vi "refnums.vi"() -> ()   [LabVIEW 2018]
panel:
  out "Wheel_1_Pot":string
  out "Wheel_4_Azimuth":string
  out "Wheel_3_Azimuth":string
  out "IMU_0":string
  out "Joystick_Driver":string
  out "Shifters":string
  out "Butterfly":string
  out "Compressor":string
  out "Wheel_2_Azimuth":string
  out "Wheel_1_Azimuth":string
  out "Wheel_4_Speed":string
  out "Wheel_3_Speed":string
  out "Wheel_2_Speed":string
  out "Wheel_1_Speed":string
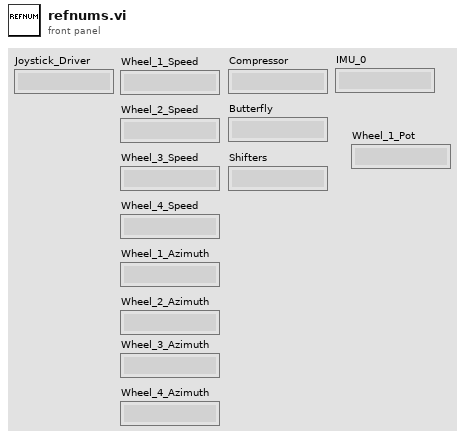
[diagram p1: front panel]
diagram:
